vi "模拟输入_电压或热电偶_连续.vi"() -> ()   [LabVIEW 2013]
doc: "本范例演示用DAQmx设备通过单个任务实现连续采集缓冲电压和热电偶测量数据的方法。一般情况下，如需对单个设备的多个通道采用不同的通道设置（测量类型、范围等），可在单个模拟输入任务中多次调用DAQmx Create Channel.vi。\n\n关于将信号连接至DAQ设备的方法，可参考设备文档。"
uses:
  <vilib>/Utility/error.llb/DialogType.ctl
  <userlib>/ArtDAQ/_SubVI/ArtDAQ_CfgSampClkTiming.vi
  <userlib>/ArtDAQ/_SubVI/ArtDAQ_CreateAIVoltageChan.vi
  <userlib>/ArtDAQ/_SubVI/ArtDAQ_CreateAIThrmcplChan.vi
  <userlib>/ArtDAQ/_SubVI/ArtDAQ_Read Analog DBL NChan NSamp.vi
panel:
  in  "停止":bool
  in  "通道设置":enum32{"Voltage", "Thermocouple"}(tab)
  in  "电压物理通道":string="Dev1/ai0" caption="物理通道"
  in  "电压最小值":dbl=-0.08 caption="最小值"
  in  "电压最大值":dbl=0.08 caption="最大值"
  in  "启用电压":bool=TRUE
  in  "接线端配置":i32(ring)=-1 items=["默认"=-1, "单端"=10083, "非参考单端"=10078, "差分"=10106, "伪差分"=12529]
  in  "热电偶物理通道":string="Dev1/ai1" caption="物理通道"
  in  "热电偶最小值":dbl caption="最小值"
  in  "热电偶最大值":dbl=100.0 caption="最大值"
  in  "单位":i32(ring)=10143 items=["Deg C"=10143, "华氏"=10144, "Kelvins"=10325, "Deg R"=10145, "来自自定义换算"=10065]
  in  "热电偶类型":i32(ring)=10072 items=["J"=10072, "k"=10073, "N"=10077, "R"=10082, "S"=10085, "T"=10086, "B"=10047, "E"=10055]
  in  "CJC源":i32(ring)=10116 items=["内置"=10200, "常量值"=10116, "通道"=10113]
  in  "CJC值":dbl=25.0
  in  "CJC通道":string
  in  "启用热电偶":bool=TRUE
  in  "每次循环采样数":i32=10
  in  "采样率":dbl=100.0
  in  "采样时钟源":string="OnboardClock"
  out "波形图":dbl[][](graph)
  # "通道设置"
  # "定时设置"
  # "采集数据"
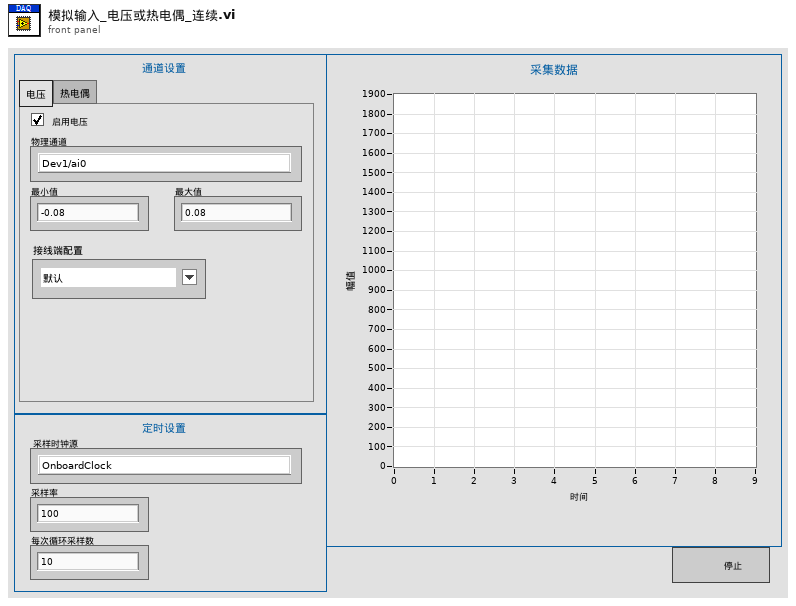
[diagram p1: front panel]
types:
  T1 = typedef "DialogType.ctl" = u16
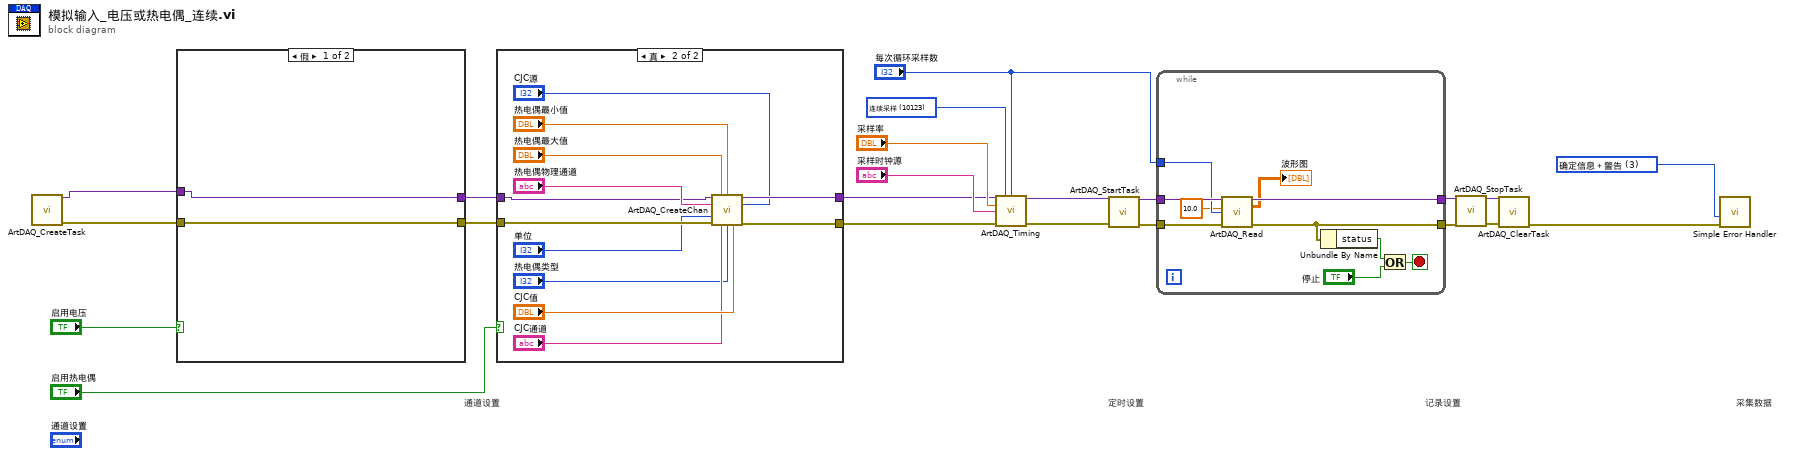
[diagram p0: block diagram]
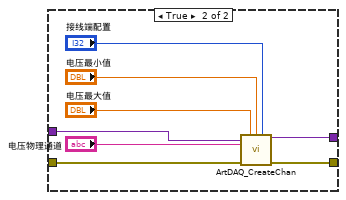
[diagram p3: hidden frame]
diagram:
  w2 = 10123 items=["有限点采样"=10178, "连续采样"=10123] ("采样模式")
  w8 = T1 3 items=["无对话框", "确定信息", "继续或停止信息", "确定信息＋警告", "继续/停止＋警告"] ("对话框类型（确定信息：1）")
  # "采集数据"
  # "定时设置"
  # "通道设置"
  # "记录设置"
  n1 = call <userlib>:"ArtDAQ_CreateTask.vi"() -> ("任务句柄"=w5:variant, "错误输出"=w4:errorcluster)  [unwired: 14 in]
  n2 = case shown="假" "启用电压" {
    tunnel: [w23 w32] -> w17
    tunnel: [w24 w31] -> w16
    tunnel: w5 -> [w24 w26]
    tunnel: w4 -> [w23 w25]
    frame False {
    }
    frame True {
      n3 = call-poly <userlib>:"ArtDAQ_CreateChan.vi"("任务句柄"=w26, "最大值"="电压最大值", "最小值"="电压最小值", "接线端配置"="接线端配置", "物理通道"="电压物理通道", "错误输入"=w25) -> ("任务句柄"=w31:variant, "错误输出"=w32:errorcluster)  [unwired: 8 in]
    }
  }
  n4 = case shown="真" "启用热电偶" {
    tunnel: [w33 w46] -> w15
    tunnel: [w34 w45] -> w3
    tunnel: w17 -> [w33 w44]
    tunnel: w16 -> [w34 w35]
    frame False {
    }
    frame True {
      n5 = call-poly <userlib>:"ArtDAQ_CreateChan.vi"("任务句柄"=w35, "最大值"="热电偶最大值", "最小值"="热电偶最小值", "物理通道"="热电偶物理通道", "CJC源"="CJC源", "单位"="单位", "错误输入"=w44, "CJC通道"="CJC通道", "热电偶类型"="热电偶类型", "CJC值"="CJC值") -> ("任务句柄"=w45:variant, "错误输出"=w46:errorcluster)  [unwired: 4 in]
    }
  }
  n6 = call-poly <userlib>:"ArtDAQ_Timing.vi"("任务句柄"=w3, "采样模式"=w2, "每通道采样数"="每次循环采样数", "采样率"="采样率", "源"="采样时钟源", "错误输入"=w15) -> ("任务句柄"=w6:variant, "错误输出"=w7:errorcluster)  [unwired: 8 in]
  n7 = call <userlib>:"ArtDAQ_StartTask.vi"("任务句柄"=w6, "错误输入"=w7) -> ("任务句柄"=w22:variant, "错误输出"=w21:errorcluster)  [unwired: 12 in]
  n8 = while {
    tunnel: w22 -> [w56]
    tunnel: w21 -> [w55]
    tunnel: [w52] -> w9
    tunnel: [w53] -> w10
    tunnel: "每次循环采样数" -> [w48]
    stop <- w54 stop-if-true
    n9 = call-poly <userlib>:"ArtDAQ_Read.vi"("任务句柄"=w56, "每通道采样数"=w48, "超时s"=10.0, "错误输入"=w55) -> ("任务句柄"=w53:variant, "数据"=→"波形图":dbl[][], "错误输出"=w52:errorcluster)  [unwired: 8 in, 1 out]
    n10 = Unbundle By Name(w52) -> ("status"=w51:bool)
    n11 = Or(x=w51, y="停止") -> (x .or. y?=w54:bool)
  }
  n12 = call <userlib>:"ArtDAQ_StopTask.vi"("任务句柄"=w10, "错误输入"=w9) -> ("任务句柄"=w12:variant, "错误输出"=w11:errorcluster)  [unwired: 12 in]
  n13 = call <userlib>:"ArtDAQ_ClearTask.vi"("任务句柄"=w12, "错误输入"=w11) -> ("错误输出"=w20:errorcluster)  [unwired: 13 in]
  n14 = call <vilib>:"Simple Error Handler.vi"("type of dialog (OK msg:1)"=w8, "error in (no error)"=w20) -> ()  [unwired: 3 in, 5 out]
